vi "Initialize Motors.vi"   [LabVIEW 2017]
uses:
  Globals/Robot Global Data.vi
types:
  T1 = typedef "WPI_MotorControlDeviceRef.ctl" = cluster{"DeviceStatus":errorcluster, "Type":T2, "PWM":cluster{"PWM Channel":T3, "DeadBand":T4}, "CAN":cluster{"Device Number":u8, "SetOutput VI Ref":variant, "GetOutput VI Ref":variant, "Enable VI Ref":variant, "Disable VI Ref":variant, "Data":variant}, "Invert":bool, "DIO PWM":cluster{"PWM \"Enable\" Channel":T3, "DIOChannel":T5, "PWM Rate":dbl}}
  T2 = typedef "WPI_MotorControlType.ctl" = enum16{"PWM", "CAN", "DIO PWM"}
  T3 = typedef "FPGA_DIOPWMChannel.ctl" = enum8{"PWM 0", "PWM 1", "PWM 2", "PWM 3", "PWM 4", "PWM 5", "PWM 6", "PWM 7", "PWM 8", "PWM 9", "PWM MXP 0", "PWM MXP 1", "PWM MXP 2", "PWM MXP 3", "PWM MXP 4", "PWM MXP 5", "PWM MXP 6", "PWM MXP 7", "PWM MXP 8", "PWM MXP 9", "Invalid"}
  T4 = typedef "WPI_PWMDeadband.ctl" = cluster{"Name":string, "maxPositivePwm":i32, "minPositivePwm":i32, "centerPwm":i32, "maxNegativePwm":i32, "minNegativePwm":i32, "angularRange":u16}
  T5 = typedef "FPGA_DIOChannel.ctl" = enum8{"DIO 0", "DIO 1", "DIO 2", "DIO 3", "DIO 4", "DIO 5", "DIO 6", "DIO 7", "DIO 8", "DIO 9", "DIO MXP 0", "DIO MXP 1", "DIO MXP 2", "DIO MXP 3", "DIO MXP 4", "DIO MXP 5", "DIO MXP 6", "DIO MXP 7", "DIO MXP 8", "DIO MXP 9", "DIO MXP 10", "DIO MXP 11", "DIO MXP 12", "DIO MXP 13", "DIO MXP 14", "DIO MXP 15", "SPI Port CS1", "SPI Port CS2", "SPI Port CS3", "SPI Port MISO", "SPI Port MOSI", "Invalid"}
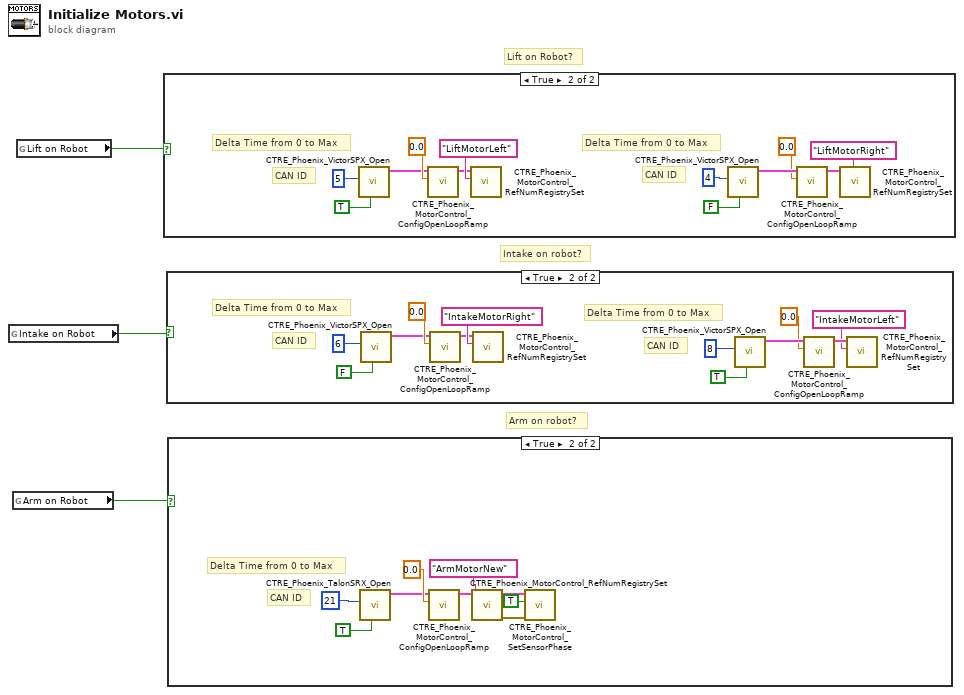
[diagram p0: block diagram]
diagram:
  # "Arm on robot?"
  # "Intake on robot?"
  # "Lift on Robot?"
  n1 = global read "Robot Global Data.vi" "Intake on Robot"() -> (w2:bool)
  n2 = global read "Robot Global Data.vi" "Arm on Robot"() -> (w1:bool)
  n3 = global read "Robot Global Data.vi" "Lift on Robot"() -> (w3:bool)
  n4 = case shown="True" w3 {
    frame False {
    }
    frame True {
      # "CAN ID"
      # "CAN ID"
      # "Delta Time from 0 to Max"
      # "Delta Time from 0 to Max"
      n5 = call "CTRE_Phoenix_VictorSPX_Open.vi"("Invert"=TRUE, "Device Number"=u8 5) -> ("CAN Talon SRX Ref"=w11:T1)  [unwired: 8 in, 1 out]
      n6 = call "CTRE_Phoenix_MotorControl_ConfigOpenLoopRamp.vi"("secondsFromNeutralToFull"=0.0, "PhoenixMotorControlDevRef"=w11) -> ("PhoenixMotorControlDevRef"=w12:T1)  [unwired: 8 in, 1 out]
      n7 = call <vilib>:"CTRE_Phoenix_MotorControl_RefNumRegistrySet.vi"("refnum name"="LiftMotorLeft", "PhoenixMotorControlDevRef"=w12) -> ()  [unwired: 8 in, 2 out]
      n8 = call "CTRE_Phoenix_VictorSPX_Open.vi"("Invert"=FALSE, "Device Number"=u8 4) -> ("CAN Talon SRX Ref"=w10:T1)  [unwired: 8 in, 1 out]
      n9 = call "CTRE_Phoenix_MotorControl_ConfigOpenLoopRamp.vi"("secondsFromNeutralToFull"=0.0, "PhoenixMotorControlDevRef"=w10) -> ("PhoenixMotorControlDevRef"=w9:T1)  [unwired: 8 in, 1 out]
      n10 = call <vilib>:"CTRE_Phoenix_MotorControl_RefNumRegistrySet.vi"("refnum name"="LiftMotorRight", "PhoenixMotorControlDevRef"=w9) -> ()  [unwired: 8 in, 2 out]
    }
  }
  n11 = case shown="True" w2 {
    frame False {
    }
    frame True {
      # "CAN ID"
      # "CAN ID"
      # "Delta Time from 0 to Max"
      # "Delta Time from 0 to Max"
      n12 = call "CTRE_Phoenix_VictorSPX_Open.vi"("Invert"=FALSE, "Device Number"=u8 6) -> ("CAN Talon SRX Ref"=w23:T1)  [unwired: 8 in, 1 out]
      n13 = call "CTRE_Phoenix_MotorControl_ConfigOpenLoopRamp.vi"("secondsFromNeutralToFull"=0.0, "PhoenixMotorControlDevRef"=w23) -> ("PhoenixMotorControlDevRef"=w24:T1)  [unwired: 8 in, 1 out]
      n14 = call <vilib>:"CTRE_Phoenix_MotorControl_RefNumRegistrySet.vi"("refnum name"="IntakeMotorRight", "PhoenixMotorControlDevRef"=w24) -> ()  [unwired: 8 in, 2 out]
      n15 = call "CTRE_Phoenix_VictorSPX_Open.vi"("Invert"=TRUE, "Device Number"=u8 8) -> ("CAN Talon SRX Ref"=w22:T1)  [unwired: 8 in, 1 out]
      n16 = call "CTRE_Phoenix_MotorControl_ConfigOpenLoopRamp.vi"("secondsFromNeutralToFull"=0.0, "PhoenixMotorControlDevRef"=w22) -> ("PhoenixMotorControlDevRef"=w21:T1)  [unwired: 8 in, 1 out]
      n17 = call <vilib>:"CTRE_Phoenix_MotorControl_RefNumRegistrySet.vi"("refnum name"="IntakeMotorLeft", "PhoenixMotorControlDevRef"=w21) -> ()  [unwired: 8 in, 2 out]
    }
  }
  n18 = case shown="True" w1 {
    frame False {
    }
    frame True {
      # "CAN ID"
      # "Delta Time from 0 to Max"
      n19 = call "CTRE_Phoenix_TalonSRX_Open.vi"("Invert"=TRUE, "Device Number"=u8 21) -> ("CAN Talon SRX Ref"=w31:T1)  [unwired: 8 in, 1 out]
      n20 = call "CTRE_Phoenix_MotorControl_ConfigOpenLoopRamp.vi"("secondsFromNeutralToFull"=0.0, "PhoenixMotorControlDevRef"=w31) -> ("PhoenixMotorControlDevRef"=w32:T1)  [unwired: 8 in, 1 out]
      n21 = call <vilib>:"CTRE_Phoenix_MotorControl_RefNumRegistrySet.vi"("refnum name"="ArmMotorNew", "PhoenixMotorControlDevRef"=w32) -> ("error out"=w30:errorcluster, "PhoenixMotorControlDevRef"=w29:T1)  [unwired: 8 in]
      n22 = call <vilib>:"CTRE_Phoenix_MotorControl_SetSensorPhase.vi"("error in (no error)"=w30, "PhaseSensor"=TRUE, "PhoenixMotorControlDevRef"=w29) -> ()  [unwired: 7 in, 2 out]
    }
  }
